vi "HS-Simulate Antenna Hardware.vi"(7 "Command to Simulate":T1, 8 "error in (no error)":errorcluster, 10 "Simulation Data":T2={"PowerOn"=TRUE, "Battery"=TRUE, "Antenna"=TRUE, "Microphone"=TRUE, "Speakers"=TRUE, "Buttons"=TRUE, "LCD"=enum."Passing Image"}, 11 "QAM Data In":cluster{dbl[], dbl[]}) -> (0 "error out":errorcluster, 3 "QAM Data Out":cluster{dbl[], dbl[]})   [LabVIEW 2019]
uses:
  Public/Documents/National Instruments/TestStand 2019 (64-bit)/Examples/Demos/Mobile Device Test/LabVIEW/Source/Support/Simulation Data.ctl
  Public/Documents/National Instruments/TestStand 2019 (64-bit)/Examples/Demos/Mobile Device Test/LabVIEW/Source/Support/Antenna Simulation States.ctl
  Public/Documents/National Instruments/TestStand 2019 (64-bit)/Examples/Demos/Mobile Device Test/LabVIEW/MobileDeviceTestDemo.llb/MobileDeviceDemo - NI_PtbyPt.lvlib
panel:
  in  "Noise":dbl(slide)=0.05 scale=0.0..0.1
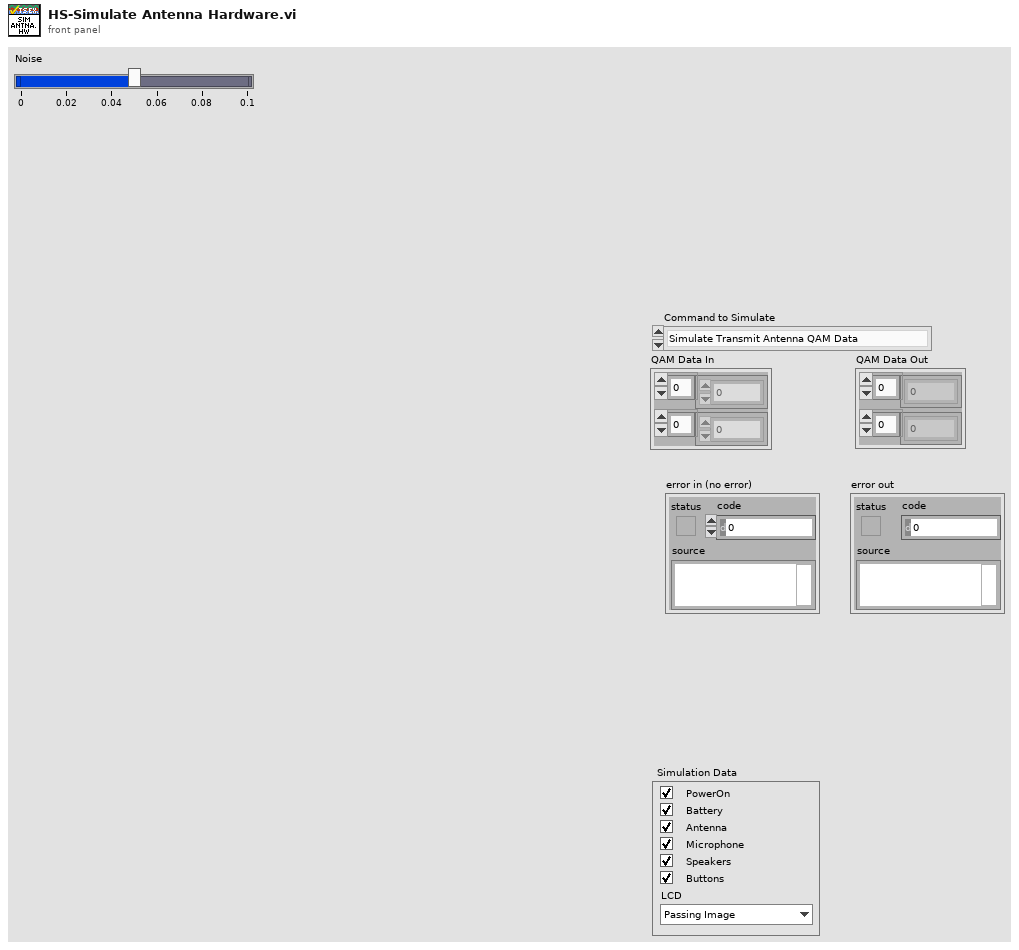
[diagram p1: front panel]
types:
  T1 = typedef "Antenna Simulation States.ctl" = enum16{"Simulate Transmit Antenna QAM Data", "Simulate Receive Antenna QAM Data"}
  T2 = typedef "Simulation Data.ctl" = cluster{"PowerOn":bool, "Battery":bool, "Antenna":bool, "Microphone":bool, "Speakers":bool, "Buttons":bool, "LCD":enum16{"Passing Image", "Dead Pixels", "Incorrect Brightness"}}
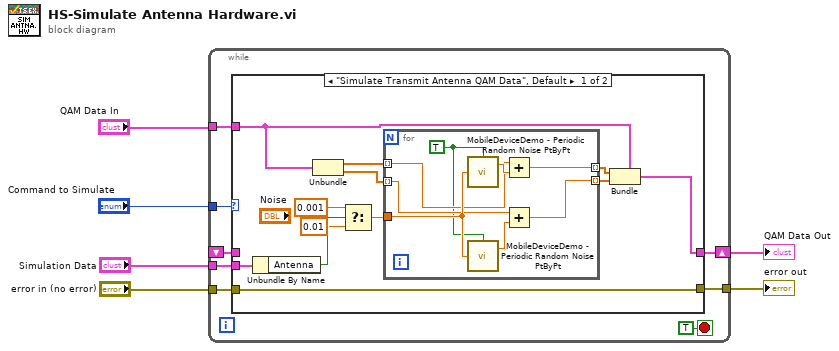
[diagram p0: block diagram]
diagram:
  n1 = while {
    tunnel: [w13] -> w6
    tunnel: "error in (no error)" -> [w12]
    tunnel: "Command to Simulate" -> [w11]
    shift-right: [w14] -> w1
    shift-left: _ -> [w10]
    tunnel: "QAM Data In" -> [w8]
    tunnel: "Simulation Data" -> [w7]
    stop <- TRUE stop-if-true
    n2 = case shown="\"Simulate Transmit Antenna QAM Data\", Default" w11 {
      tunnel: [w19 w36] -> w14
      tunnel: [w25 w35] -> w13
      tunnel: w12 -> [w25 w35]
      tunnel: w10 -> [_ w36]
      tunnel: w8 -> [w22 _]
      tunnel: w7 -> [w26 _]
      frame "Simulate Transmit Antenna QAM Data", Default {
        n3 = Unbundle By Name(w26) -> ("Antenna"=w17:bool)
        n4 = Unbundle(w22) -> (w24:dbl[], w23:dbl[])
        n5 = Select(t=0.001, s=w17, f=0.01) -> (s? t:f=w18:dbl)
        n6 = for {
          tunnel: w18 -> [w32]
          tunnel: w24 -> [w31] mode=indexing
          tunnel: w23 -> [w30] mode=indexing
          tunnel: [w29] -> w21 mode=indexing
          tunnel: [w28] -> w20 mode=indexing
          w27 = TRUE ("initialize")
          n7 = call "MobileDeviceDemo - Periodic Random Noise PtByPt.vi"("initialize"=w27, "spectral amplitude"=w32) -> ("periodic random noise"=w33:dbl)  [unwired: 2 in, 1 out]
          n8 = call "MobileDeviceDemo - Periodic Random Noise PtByPt.vi"("initialize"=w27, "spectral amplitude"=w32) -> ("periodic random noise"=w34:dbl)  [unwired: 2 in, 1 out]
          n9 = Add(x=w31, y=w33) -> (x+y=w29:dbl)
          n10 = Add(x=w30, y=w34) -> (x+y=w28:dbl)
        }
        n11 = Bundle(cluster=w22, w21, w20) -> (w19:cluster{dbl[], dbl[]})
      }
      frame "Simulate Receive Antenna QAM Data" {
      }
    }
  }
  "error out" <- w6
  "QAM Data Out" <- w1
